vi "n64_shape_single_axis.vi"(10 "Row Length":i32=8, 11 "Readings (FLAT)":dbl[](array[numeric])) -> (3 "Readings (GRID)":dbl[][](array[numeric]))   [LabVIEW 2016]
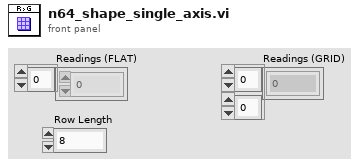
[diagram p1: front panel]
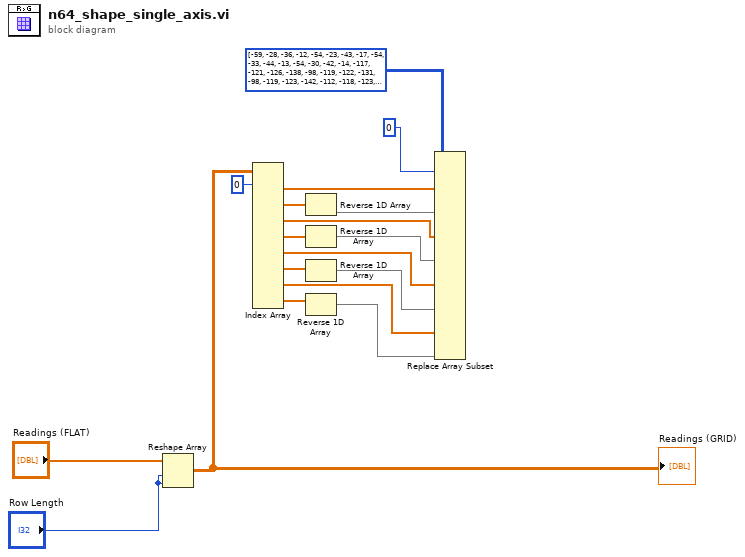
[diagram p0: block diagram]
diagram:
  n1 = Reshape Array("Readings (FLAT)", "Row Length", "Row Length") -> (w1:dbl[][])
  "Readings (GRID)" <- w1
  n2 = Index Array(array=w1, index (row) #1=0 ("index (row)")) -> (element #1=w12:dbl[], element #2=w17:dbl[], element #3=w7:dbl[], element #4=w16:dbl[], element #5=w5:dbl[], element #6=w15:dbl[], element #7=w3:dbl[], element #8=w14:dbl[])  [unwired: 15 in]
  n3 = Reverse 1D Array(array=w17) -> (reversed array=w8:dbl[])
  n4 = Reverse 1D Array(array=w16) -> (reversed array=w6:dbl[])
  n5 = Reverse 1D Array(array=w15) -> (reversed array=w4:dbl[])
  n6 = Reverse 1D Array(array=w14) -> (reversed array=w2:dbl[])
  n7 = Replace Array Subset(array=i16[][] [[-59, -28, -36, -12, -54, -23, -43, -17], [-54, -33, -44, -13, -54, -30, -42, -14], [-117, -121, -126, -138, -98, -119, -122, -131], [-98, -119, -123, -142, -112, -118, -123, -142], [-29, 11, 96, 200, -26, 12, 97, 205], [-14, 9, 92, 199, -27, 14, 103, 193], [-63, -15, 69, 356, -74, -25, 54, 362], [-70, -22, 65, 350, -65, -28, 58, 359]] ("reshaped"), new element #1=w12, index (row) #1=0 ("index (row)"), new element #2=w8, new element #3=w7, new element #4=w6, new element #5=w5, new element #6=w4, new element #7=w3, new element #8=w2) -> ()  [unwired: 15 in, 1 out]
